vi "Distend (DBL).vi"(6 "Distend method":T1=enum."Linear distance from center", 7 "Weighting":dbl[](graph), 9 "Keep silhuette size?(F)":bool, 10 "Distend":dbl, 11 "X":dbl[](graph)) -> (3 "X Distended":dbl[](graph))   [LabVIEW 2015, in "Morph Cortical Surfaces.lvlib"]
doc: "Distends values such, that values near the median are not changed much, and values near max and min are changed up to Distend value. The function is exponential in shape. With False as Keep silhuette size positive Distend values increase the size, negative decrease. With T only the shape will change but the max and min values will be the same."
uses:
  Morph Cortical Surfaces.lvlib
  Distend method control.ctl
  <vilib>/Analysis/NI_AALBase.lvlib
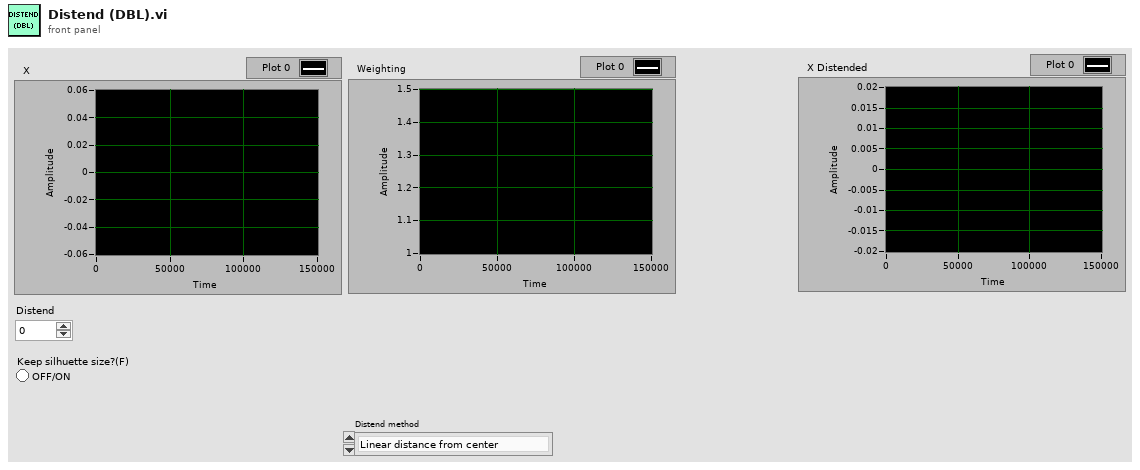
[diagram p1: front panel]
types:
  T1 = typedef "Morph Cortical Surfaces.lvlib/Distend method control.ctl" = enum16{"Use weighting values", "Linear distance from center", "Exponential distance from center"}
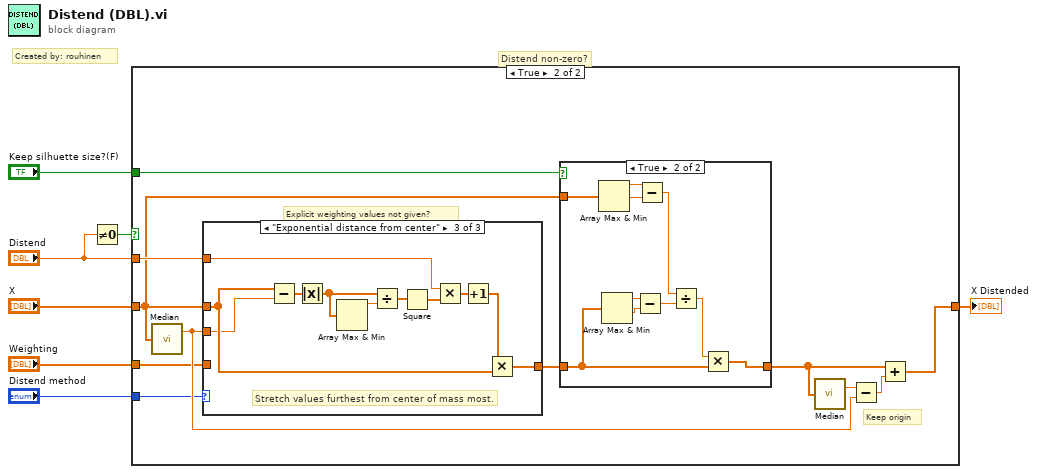
[diagram p0: block diagram]
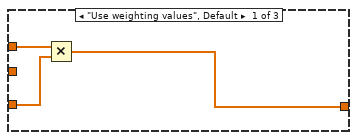
[diagram p3: hidden frame]
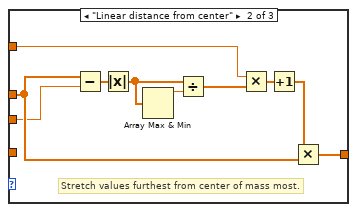
[diagram p4: hidden frame]
diagram:
  # "Created by: rouhinen"
  # "Distend non-zero?"
  n1 = Not Equal To 0?(x="Distend") -> (x != 0?=w6:bool)
  n2 = case shown="True" w6 {
    tunnel: "Distend" -> [_ w19]
    tunnel: [w8 w16] -> w2
    tunnel: "X" -> [w8 w12]
    tunnel: "Keep silhuette size?(F)" -> [_ w17]
    tunnel: "Weighting" -> [_ w10]
    tunnel: "Distend method" -> [_ w9]
    frame False {
    }
    frame True {
      # "Explicit weighting values not given?"
      # "Keep origin"
      n3 = call <vilib>:"Median.vi"("X"=w12) -> ("median"=w11:dbl)  [unwired: 1 out]
      n4 = case shown="\"Exponential distance from center\"" w9 {
        tunnel: w19 -> [_ w29 w40]
        tunnel: [w20 w26 w37] -> w18
        tunnel: w12 -> [w21 w25 w36]
        tunnel: w11 -> [_ w24 w35]
        tunnel: w10 -> [w22 _ _]
        frame "Use weighting values", Default {
          n5 = Multiply(x=w21, y=w22) -> (x*y=w20:dbl[])
        }
        frame "Linear distance from center" {
          # "Stretch values furthest from center of mass most."
          n6 = Subtract(x=w25, y=w24) -> (x-y=w32:dbl[])
          n7 = Absolute Value(x=w32) -> (abs(x)=w30:dbl[])
          n8 = Array Max & Min(array=w30) -> (max value=w31:dbl)  [unwired: 3 out]
          n9 = Divide(x=w30, y=w31) -> (x/y=w23:dbl[])
          n10 = Multiply(x=w29, y=w23) -> (x*y=w28:dbl[])
          n11 = Increment(x=w28) -> (x+1=w27:dbl[])
          n12 = Multiply(x=w27, y=w25) -> (x*y=w26:dbl[])
        }
        frame "Exponential distance from center" {
          # "Stretch values furthest from center of mass most."
          n13 = Subtract(x=w36, y=w35) -> (x-y=w43:dbl[])
          n14 = Absolute Value(x=w43) -> (abs(x)=w41:dbl[])
          n15 = Array Max & Min(array=w41) -> (max value=w42:dbl)  [unwired: 3 out]
          n16 = Divide(x=w41, y=w42) -> (x/y=w34:dbl[])
          n17 = Square(x=w34) -> (x^2=w33:dbl[])
          n18 = Multiply(x=w40, y=w33) -> (x*y=w39:dbl[])
          n19 = Increment(x=w39) -> (x+1=w38:dbl[])
          n20 = Multiply(x=w38, y=w36) -> (x*y=w37:dbl[])
        }
      }
      n21 = case shown="True" w17 {
        tunnel: w12 -> [_ w54]
        tunnel: w18 -> [w44 w47]
        tunnel: [w44 w45] -> w15
        frame False {
        }
        frame True {
          n22 = Array Max & Min(array=w54) -> (max value=w53:dbl, min value=w52:dbl)  [unwired: 2 out]
          n23 = Array Max & Min(array=w47) -> (max value=w51:dbl, min value=w50:dbl)  [unwired: 2 out]
          n24 = Subtract(x=w51, y=w50) -> (x-y=w49:dbl)
          n25 = Subtract(x=w53, y=w52) -> (x-y=w48:dbl)
          n26 = Divide(x=w48, y=w49) -> (x/y=w46:dbl)
          n27 = Multiply(x=w46, y=w47) -> (x*y=w45:dbl[])
        }
      }
      n28 = call <vilib>:"Median.vi"("X"=w15) -> ("median"=w14:dbl)  [unwired: 1 out]
      n29 = Subtract(x=w14, y=w11) -> (x-y=w13:dbl)
      n30 = Add(x=w15, y=w13) -> (x+y=w16:dbl[])
    }
  }
  "X Distended" <- w2
